vi "Draw.vi"(8 "error in (no error)":errorcluster, 10 "2D Picture in":picture, 11 "Triangle in":refnum<class "Losange.lvclass">) -> (0 "error out":errorcluster, 2 "2D Picture out":picture, 3 "Triangle out":refnum<class "Losange.lvclass">)   [LabVIEW 2021, in "Picture2D.lvlib" / "Losange.lvclass"]
uses:
  Losange.lvclass
  Losange.lvclass/Losange.ctl
  Polygone/Polygone.lvclass
  Color/Color.lvclass
  Point/Point.lvclass
  Pen/Pen.lvclass
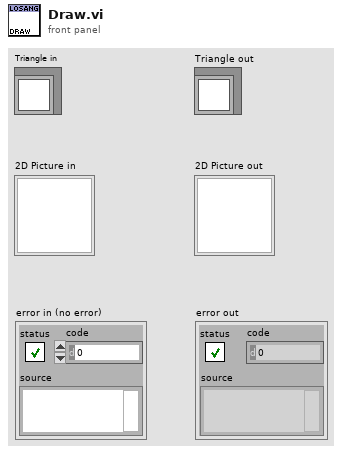
[diagram p1: front panel]
types:
  T1 = cluster{"Width":u16, "Style":enum32{"Solid", "Dash", "Dot", "DashDot", "DashDotDot"}}
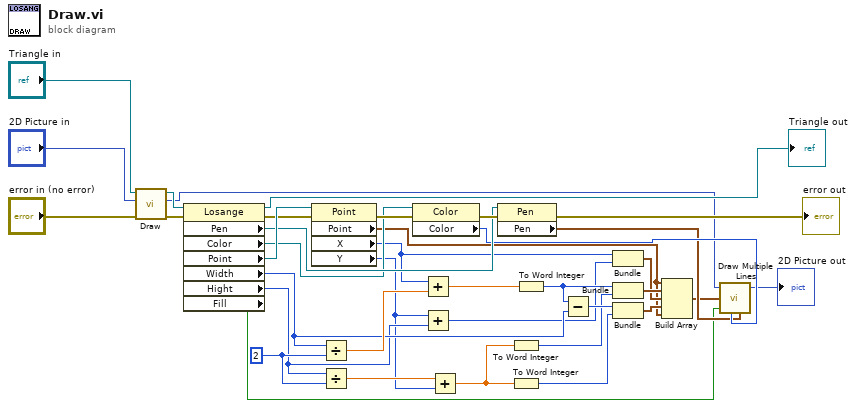
[diagram p0: block diagram]
diagram:
  w18 = i16 2 ("y")
  n1 = call-parent "Draw.vi"("error in (no error)"="error in (no error)", "2D Picture in"="2D Picture in", "Shape in"="Triangle in") -> ("error out"=w27:errorcluster, "2D Picture out"=w2:picture, "Shape out"=w34:refnum<class "Losange.lvclass">)  [unwired: 6 in]
  n2 = property class="Losange"(reference=w34, error in=w27) -> (reference out=→"Triangle out":refnum<class "Losange.lvclass">, error out=w30:errorcluster, "Pen"=w24:refnum<class "Pen.lvclass">, "Color"=w23:refnum<class "Color.lvclass">, "Point"=w33:refnum<class "Point.lvclass">, "Width"=w20:i16, "Hight"=w16:i16, "Fill"=w1:bool)
  n3 = property class="Point"(reference=w33, error in=w30) -> (error out=w29:errorcluster, "Point"=w4:cluster{"x":i16, "y":i16}, "X"=w13:i16, "Y"=w15:i16)  [unwired: 1 out]
  n4 = Divide(x=w20, y=w18) -> (x/y=w32:dbl)
  n5 = Divide(x=w16, y=w18) -> (x/y=w17:dbl)
  n6 = property class="Color"(reference=w23, error in=w29) -> (error out=w28:errorcluster, "Color"=w10:u32)  [unwired: 1 out]
  n7 = Add(x=w13, y=w32) -> (x+y=w31:dbl)
  n8 = Add(x=w15, y=w16) -> (x+y=w14:i16)
  n9 = Add(x=w17, y=w15) -> (x+y=w22:dbl)
  n10 = property class="Pen"(reference=w24, error in=w28) -> (error out=→"error out":errorcluster, "Pen"=w9:T1)  [unwired: 1 out]
  n11 = To Word Integer(number=w22) -> (16bit integer=w12:i16)
  n12 = To Word Integer(number=w22) -> (16bit integer=w11:i16)
  n13 = To Word Integer(number=w31) -> (16bit integer=w21:i16)
  n14 = Subtract(x=w21, y=w20) -> (x-y=w19:i16)
  n15 = Bundle("X"=w13, w14) -> (w6:cluster{"X":i16, i16})  [unwired: 1 in]
  n16 = Bundle(w21, w12) -> (w7:cluster{i16, i16})  [unwired: 1 in]
  n17 = Bundle(w19, w11) -> (w5:cluster{i16, i16})  [unwired: 1 in]
  n18 = Build Array(w4, w7, w6, w5, w4) -> (w3:cluster{"x":i16, "y":i16}[])
  n19 = call <vilib>:"Draw Multiple Lines.vi"("picture"=w2, "line endpoints"=w3, "fill?(F)"=w1, "color(black)"=w10, "pen"=w9) -> ("new picture"=→"2D Picture out":picture)  [unwired: 4 in]
